vi "Add texture.vi"(10 "Image":T1, 11 "Scene.Object In":refnum<vi>) -> (3 "Scene.Object Out":refnum<vi>)   [LabVIEW 2019]
uses:
  <vilib>/picture/picture.llb/imagedata.ctl
  <vilib>/picture/3D Picture Control/NI_3D Picture Control.lvlib
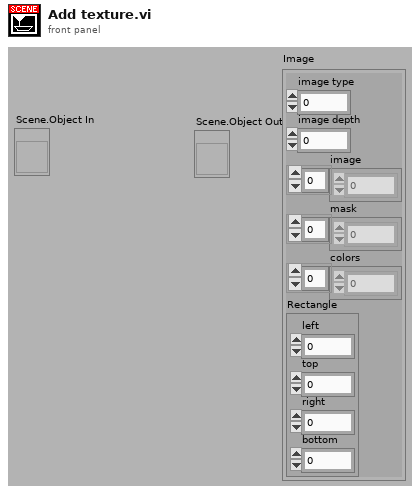
[diagram p1: front panel]
types:
  T1 = typedef "imagedata.ctl" = cluster{"image type":i32, "image depth":i32, "image":u8[], "mask":u8[], "colors":u32[], "Rectangle":cluster{"left":i16, "top":i16, "right":i16, "bottom":i16}}
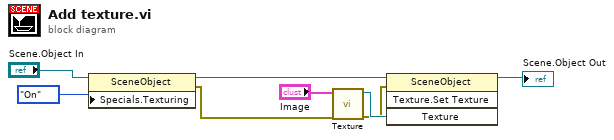
[diagram p0: block diagram]
diagram:
  n1 = property class="SceneObject"(reference="Scene.Object In", "Specials.Texturing"=enum16{"Inherit Value", "Off", "On"}."On" ("Specials:Texturing")) -> (reference out=w5:refnum<vi>, error out=w2:errorcluster)  [unwired: 1 in]
  n2 = call <vilib>:"Texture.vi"("error in (no error)"=w2, "Image"="Image") -> ("error out"=w3:errorcluster, "New Texture Refnum"=w4:refnum<vi>)  [unwired: 8 in]
  n3 = invoke class="SceneObject" method="Texture.Set Texture"(reference=w5, error in=w3, "Texture"=w4) -> (reference out=→"Scene.Object Out":refnum<vi>)  [unwired: 1 in, 3 out]
